vi "Example Callback - Current Callback.vi"(4 "Current":refnum<user-event>, 5 "Event Data":T1, 6 "Control Ref":refnum<k24>, 7 "Event Common Data":T2) -> ()   [LabVIEW 2010]
uses:
  C:/tf/play/labview/Tinkerforge.dll
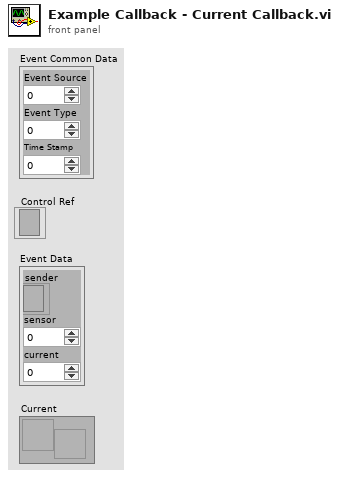
[diagram p1: front panel]
types:
  T1 = cluster{"sender":refnum<k24>, "sensor":u8, "current":i32}
  T2 = cluster{"Event Source":i32, "Event Type":u32, "Time Stamp":u32}
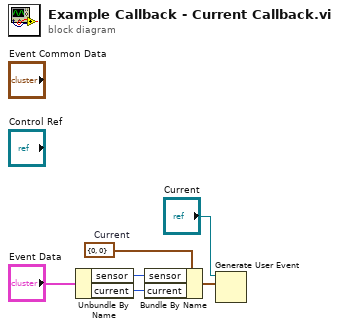
[diagram p0: block diagram]
diagram:
  w5 = cluster{"sensor":u8, "current":i32} {"sensor"=0, "current"=0}  # Current
  n1 = Unbundle By Name("Event Data") -> ("sensor"=w4:u8, "current"=w3:i32)
  n2 = Bundle By Name(cluster=w5, "sensor"=w4, "current"=w3) -> (w2:cluster{"sensor":u8, "current":i32})
  n3 = Generate User Event(user event="Current", event data cluster=w2) -> ()  [unwired: 1 in, 2 out]
